vi "ChannelToDeviceAddress.vi"(11 "InputChannel":i16) -> (2 "MotorNumber":i16, 3 "DeviceAddress":i16)   [LabVIEW 2020]
panel:
  out "Quotient":i16
  out "Remainder":i16
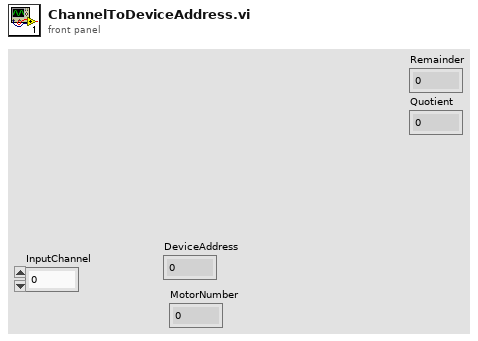
[diagram p1: front panel]
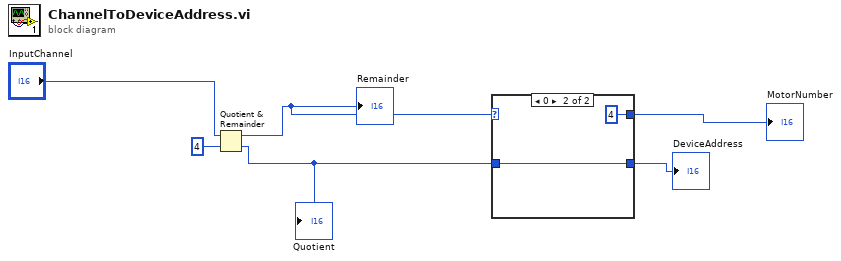
[diagram p0: block diagram]
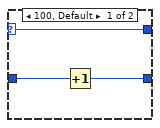
[diagram p2: hidden frame]
diagram:
  n1 = Quotient & Remainder(x="InputChannel", y=i16 4) -> (x-y*floor(x/y)=w5:i16, floor(x/y)=w3:i16)
  "Remainder" <- w5
  "Quotient" <- w3
  n2 = case shown="0" w5 {
    selector: w5 -> [w9 _]
    tunnel: [w9 i16 4] -> w4
    tunnel: w3 -> [w8 w10]
    tunnel: [w7 w10] -> w2
    frame 100, Default {
      n3 = Increment(x=w8) -> (x+1=w7:i16)
    }
    frame 0 {
    }
  }
  "DeviceAddress" <- w2
  "MotorNumber" <- w4
